vi "ReadValueByMarker.vi"(8 "error in (no error)":errorcluster, 10 "ValueMarker":string, 11 "Arduino in":refnum<class "Arduino.lvclass">) -> (0 "error out":errorcluster, 2 "ValueOut":i32, 3 "Arduino out":refnum<class "Arduino.lvclass">)   [LabVIEW 2013, in "Arduino.lvclass"]
uses:
  Arduino.lvclass
  <vilib>/regexp/Match Regular Expression.xnode
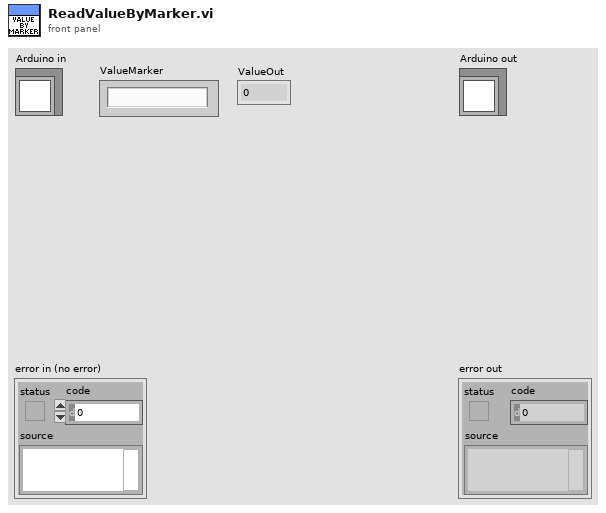
[diagram p1: front panel]
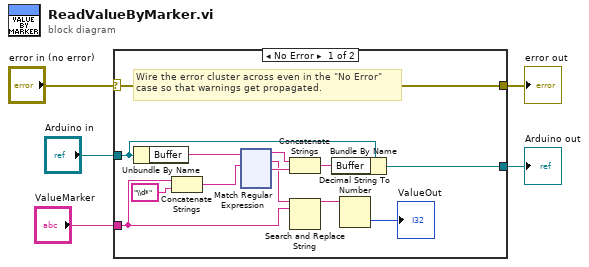
[diagram p0: block diagram]
diagram:
  n1 = case shown="No Error" "error in (no error)" {
    selector: "error in (no error)" -> [w18 w134]
    tunnel: [w18 w134] -> w4
    tunnel: [w6 w133] -> w2
    tunnel: "Arduino in" -> [w7 w133]
    tunnel: "ValueMarker" -> [w11 _]
    frame No Error {
      # "Wire the error cluster across even in the \"No Error\"\ncase so that warnings get propagated."
      n2 = Unbundle By Name(w7) -> ("Buffer"=w9:string)
      n3 = Concatenate Strings(w11, "\\d*") -> (w16:string)
      n4 = xnode "Match Regular Expression"("input string"=w9, "regular expression"=w16) -> ("before match"=w15:string, "whole match"=w12:string, "after match"=w14:string)  [unwired: 4 in, 2 out]
      n5 = Concatenate Strings(w15, w14) -> (w8:string)
      n6 = Search and Replace String(input string=w12, search string=w11) -> (result string=w10:string)  [unwired: 6 in, 3 out]
      n7 = Bundle By Name(cluster=w7, "Buffer"=w8) -> (w6:refnum<class "Arduino.lvclass">)
      n8 = Decimal String To Number(string=w10) -> (number=→"ValueOut":i32)  [unwired: 2 in, 1 out]
    }
    frame Error {
    }
  }
  "error out" <- w4
  "Arduino out" <- w2
